vi "SaveStatMeas.vi"(4 "Temp":dbl, 5 "Min":dbl, 6 "Max":dbl, 7 "error in":errorcluster, 8 "Ecart Type":dbl, 9 "Moyenne":dbl, 10 "storage refnum (file)":refnum<k20>) -> (0 "error out":errorcluster, 2 "storage refnum (file) 2":refnum<k20>)   [LabVIEW 2014]
uses:
  <vilib>/Platform/storage/Storage.llb/usiSequenceRepresentation.ctl
  <vilib>/Platform/storage/Storage.llb/usiOverwriteOptions.ctl
  <vilib>/Platform/storage/lvStorage.llb/_createOrGetByNameExplicitChildObject.vi
  <vilib>/Platform/storage/Storage.llb/__savePropString.vi
  <vilib>/Platform/storage/lvStorage.llb/xStorage/xStorageSupp/ErrorOut.vi
  <vilib>/Platform/storage/lvStorage.llb/__saveFloat64Channel.vi
  <vilib>/Platform/storage/lvStorage.llb/xStorage/Write Data/Write Data.xnode
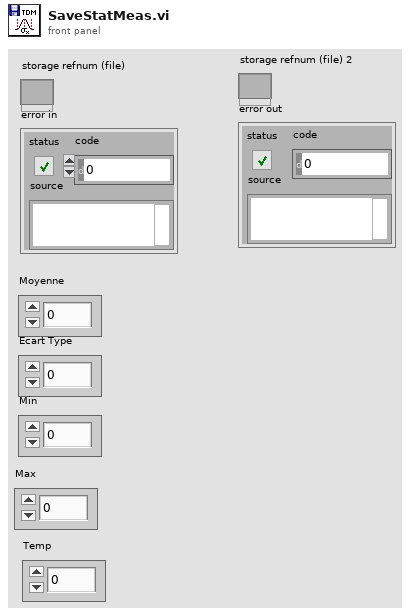
[diagram p1: front panel]
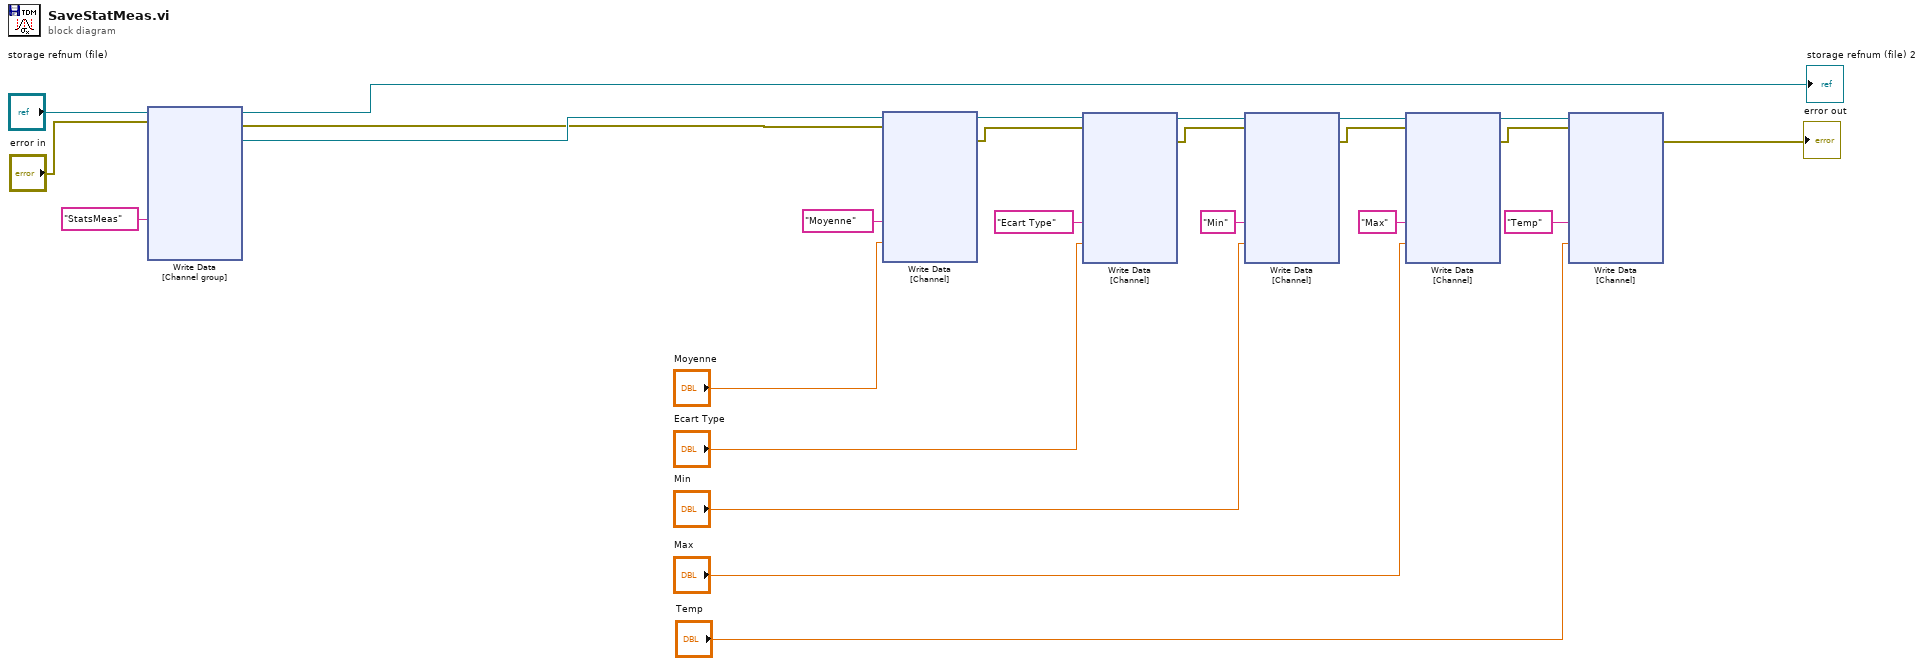
[diagram p0: block diagram]
diagram:
  n1 = xnode "Write Data\n[Channel group]"("Name"="StatsMeas", "storage refnum (file)"="storage refnum (file)", "error in"="error in") -> ("error out"=w21:errorcluster, "storage refnum (channel group)"=w22:refnum<k20>)  [unwired: 1 in, 1 out]
  n2 = xnode "Write Data\n[Channel]"("Name"="Moyenne", "Signal"="Moyenne", "storage refnum (channel group)"=w22, "error in"=w21) -> ("storage refnum (channel group) out"=w15:refnum<k20>, "error out"=w18:errorcluster)  [unwired: 2 in, 1 out]
  n3 = xnode "Write Data\n[Channel]"("Name"="Ecart Type", "Signal"="Ecart Type", "storage refnum (channel group)"=w15, "error in"=w18) -> ("storage refnum (channel group) out"=w14:refnum<k20>, "error out"=w13:errorcluster)  [unwired: 2 in, 1 out]
  n4 = xnode "Write Data\n[Channel]"("Name"="Min", "Signal"="Min", "storage refnum (channel group)"=w14, "error in"=w13) -> ("storage refnum (channel group) out"=w8:refnum<k20>, "error out"=w7:errorcluster)  [unwired: 2 in, 1 out]
  n5 = xnode "Write Data\n[Channel]"("Name"="Max", "Signal"="Max", "storage refnum (channel group)"=w8, "error in"=w7) -> ("storage refnum (channel group) out"=w5:refnum<k20>, "error out"=w4:errorcluster)  [unwired: 2 in, 1 out]
  n6 = xnode "Write Data\n[Channel]"("Name"="Temp", "Signal"="Temp", "storage refnum (channel group)"=w5, "error in"=w4) -> ("error out"=→"error out":errorcluster)  [unwired: 2 in, 2 out]
  "storage refnum (file) 2" <- "storage refnum (file)"
